vi "OAT Easy Resample Order Tracking.vi"   [LabVIEW 2017]
doc: "Computes magnitudes and phase lags for the designated orders for <B>scaled signal [EU]</B>. You can use this polymorphic VI to perform order tracking with resampling for an analog tachometer signal or a digital tachometer signal. The data type you wire to the <B>analog tach signal</B> input determines the polymorphic instance to use."
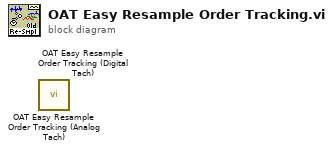
[diagram p0: block diagram]
diagram:
  n1 = call <vilib>:"OAT Easy Resample Order Tracking (Analog Tach).vi"() -> ()  [unwired: 11 in, 5 out]
  n2 = call <vilib>:"OAT Easy Resample Order Tracking (Digital Tach).vi"() -> ()  [unwired: 11 in, 5 out]
